vi "chart axis set minor tick mark.vi"(8 "error in (no error)":errorcluster, 10 "type":u8, 11 "axis":u32) -> (0 "error out":errorcluster)   [LabVIEW 8.6]
doc: "void chart_axis_set_minor_tick_mark(lxw_chart_axis axis, uint8_t type);"
uses:
  pending_lvxlsxwriter/xlsxwriter.dll
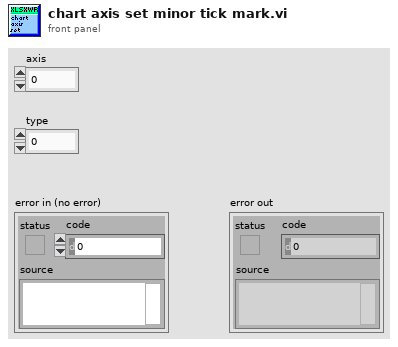
[diagram p1: front panel]
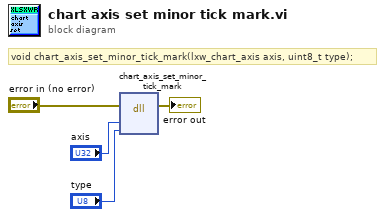
[diagram p0: block diagram]
diagram:
  # "void chart_axis_set_minor_tick_mark(lxw_chart_axis axis, uint8_t type);"
  n1 = dll-call lib="C:/Users/WDAGUtilityAccount/Desktop/pending_lvxlsxwriter/xlsxwriter.*" fn="chart_axis_set_minor_tick_mark"(error in="error in (no error)", "axis"="axis", "type"="type") -> (error out=→"error out":errorcluster)  [unwired: 5 in, 1 out]
